vi "Write Gauge Refnum.vi"(10 "Gauge Refnum":refnum<vi>, 11 "Simple Actor in":refnum<class "Simple Actor.lvclass">) -> (3 "Simple Actor out":refnum<class "Simple Actor.lvclass">)   [LabVIEW 2012, in "Simple Actor.lvclass"]
uses:
  Simple Actor.lvclass
  Simple Actor.lvclass/Simple Actor.ctl
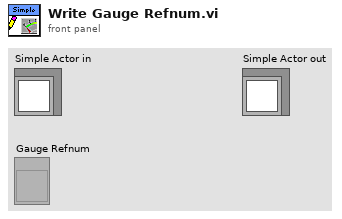
[diagram p1: front panel]
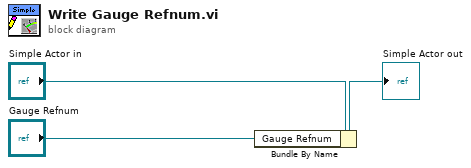
[diagram p0: block diagram]
diagram:
  n1 = Bundle By Name(cluster="Simple Actor in", "Gauge Refnum"="Gauge Refnum") -> (→"Simple Actor out":refnum<class "Simple Actor.lvclass">)
